vi "Is URI Relative.vi"(5 "URI":string="ws://hostname.domain:80/resource/name") -> (6 "URI Out":string="ws://hostname.domain:80/resource/name", 10 "Relative":bool)   [LabVIEW 2016, in "WebSockets.lvlib"]
uses:
  WebSockets.lvlib
  <vilib>/regexp/Match Regular Expression.xnode
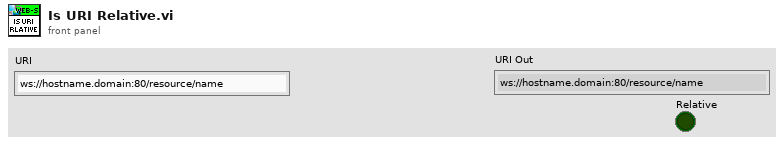
[diagram p1: front panel]
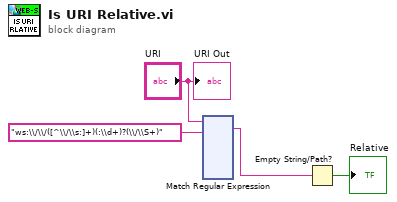
[diagram p0: block diagram]
diagram:
  n1 = xnode "Match Regular Expression"("input string"="URI", "regular expression"="ws:\\/\\/([^\\/\\s:]+)(:\\d+)?(\\/\\S+)") -> ("whole match"=w2:string)  [unwired: 4 in, 7 out]
  n2 = Empty String/Path?(string/path=w2) -> (empty?=→"Relative":bool)
  "URI Out" <- "URI"
